vi "pump calibration.vi"(4 "pump ID":u8, 6 "pump cal command":T3=enum."Save default values", 8 "STAMP intercept":dbl, 9 "STAMP slope":dbl=2.52, 10 "flow rate":dbl[unit], 11 "Pump Calibration in":T1={"target 1"=0.0, "target 2"=0.0, "measured 1"=1e-06, "measured 2"=1e-06}) -> (0 "STAMP intercept out":dbl, 1 "STAMP slope out":dbl=2.52, 2 "modified flow rate":dbl[unit], 3 "Pump Calibration out":T1)   [LabVIEW 2010]
uses:
  calibration values.ctl
  calibration commands.ctl
  <vilib>/Utility/config.llb/Write Key (Double).vi
  <vilib>/Utility/config.llb/Read Key (Double).vi
  <vilib>/Utility/config.llb/NI_LVConfig.lvlib
panel:
  in  "pump calibrations default":T2(array[cluster])=[{"Pump Calibration"={"target 1"=0.0, "target 2"=1e-06, "measured 1"=0.0, "measured 2"=1e-06}, "STAMP slope"=1.0, "STAMP intercept"=0.0}, {"Pump Calibration"={"target 1"=0.0, "target 2"=1e-06, "measured 1"=0.0, "measured 2"=0.0}, "STAMP slope"=1.0, "STAMP intercept"=0.0}, {"Pump Calibration"={"target 1"=0.0, "target 2"=1e-06, "measured 1"=0.0, "measured 2"=0.0}, "STAMP slope"=1.0, "STAMP intercept"=0.0}, {"Pump Calibration"={"target 1"=0.0, "target 2"=1e-06, "measured 1"=0.0, "measured 2"=0.0}, "STAMP slope"=1.0, "STAMP intercept"=0.0}, {"Pump Calibration"={"target 1"=0.0, "target 2"=1e-06, "measured 1"=0.0, "measured 2"=0.0}, "STAMP slope"=1.0, "STAMP intercept"=0.0}, {"Pump Calibration"={"target 1"=0.0, "target 2"=1e-06, "measured 1"=0.0, "measured 2"=0.0}, "STAMP slope"=1.0, "STAMP intercept"=0.0}]
  out "pump calibrations":T2(array[cluster])
  in  "Pump Calibration default":T1={"target 1"=0.0, "target 2"=1e-06, "measured 1"=0.0, "measured 2"=1e-06}
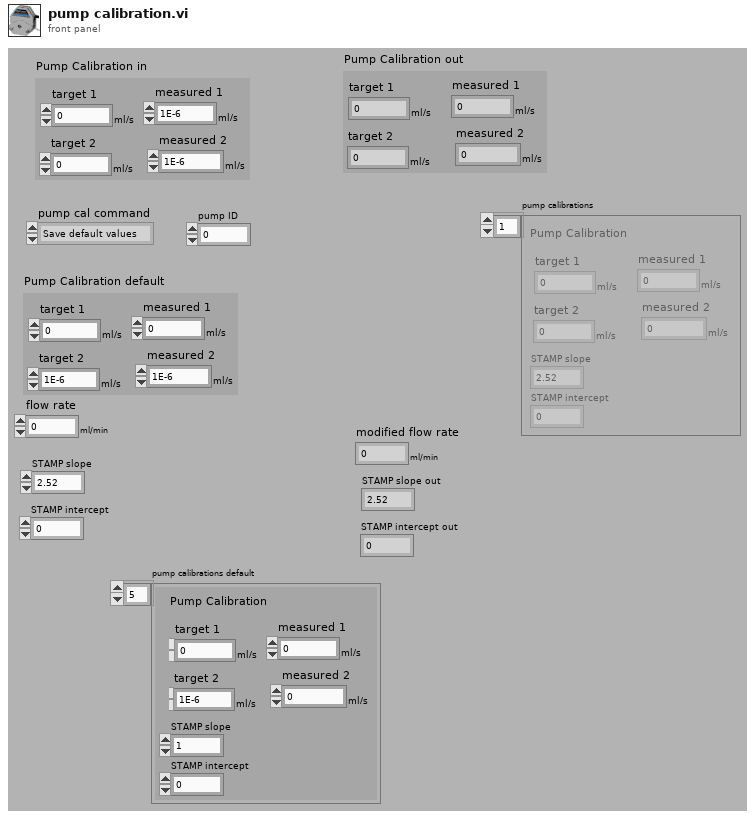
[diagram p1: front panel]
types:
  T1 = typedef "calibration values.ctl" = cluster{"target 1":dbl[unit], "target 2":dbl[unit], "measured 1":dbl[unit], "measured 2":dbl[unit]}
  T2 = cluster{"Pump Calibration":T1, "STAMP slope":dbl, "STAMP intercept":dbl}[]
  T3 = typedef "calibration commands.ctl" = enum16{"Get ini Path", "Save default values", "Save new calibration", "Read calibration", "Apply calibration", "Read STAMP mb", "Write STAMP mb"}
  T4 = typedef "NI_LVConfig.lvlib/Config Data RefNum.ctl" = refnum<k1>
  T5 = cluster{"Pump Calibration":T1, "STAMP slope":dbl, "STAMP intercept":dbl}
  T6 = cluster{"[0]":dbl[unit], "[1]":dbl[unit], "[2]":dbl[unit], "[3]":dbl[unit]}
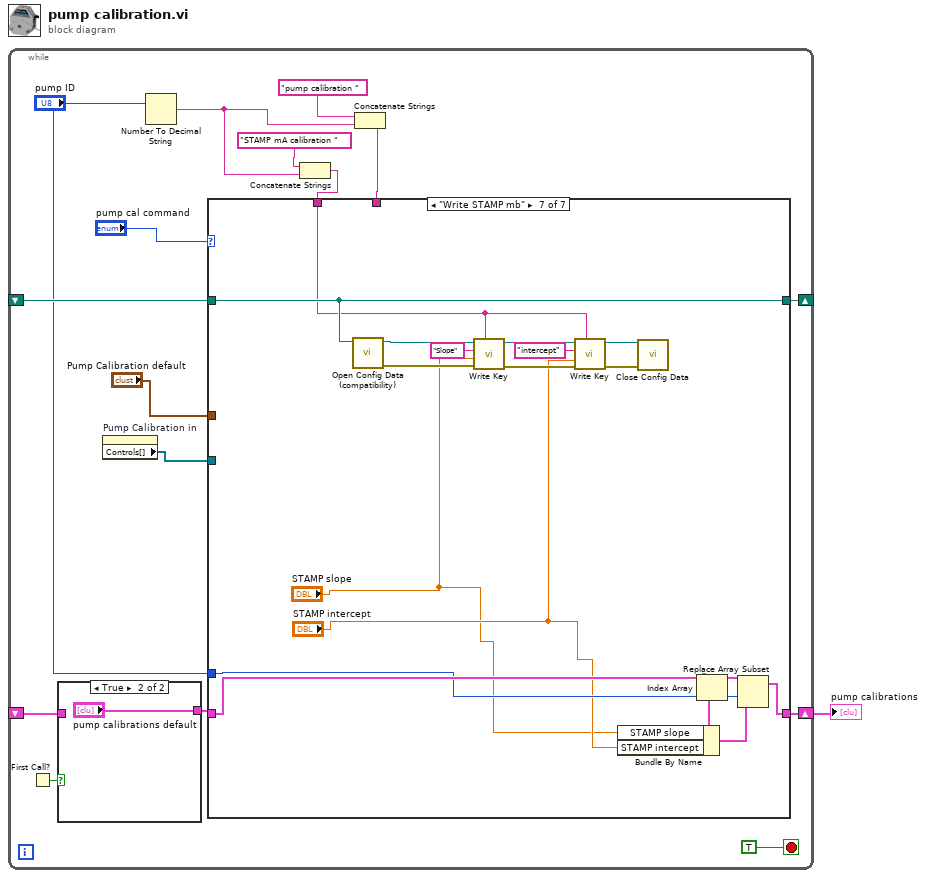
[diagram p0: block diagram]
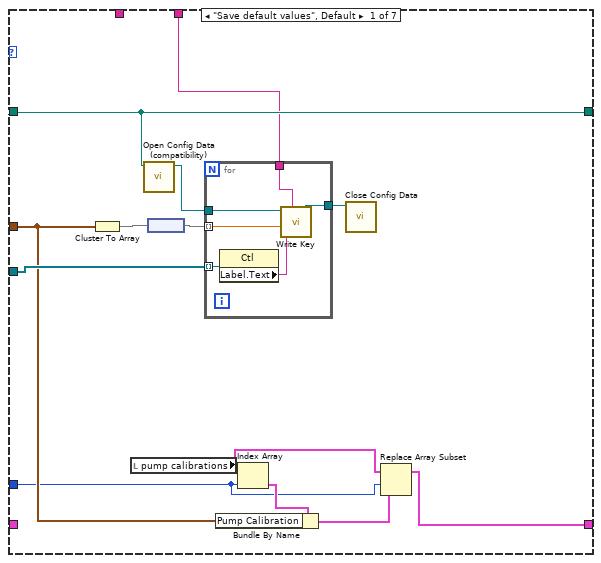
[diagram p3: hidden frame]
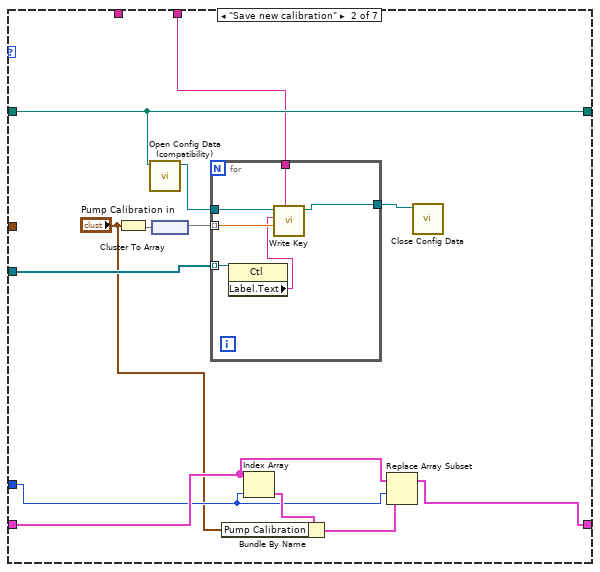
[diagram p4: hidden frame]
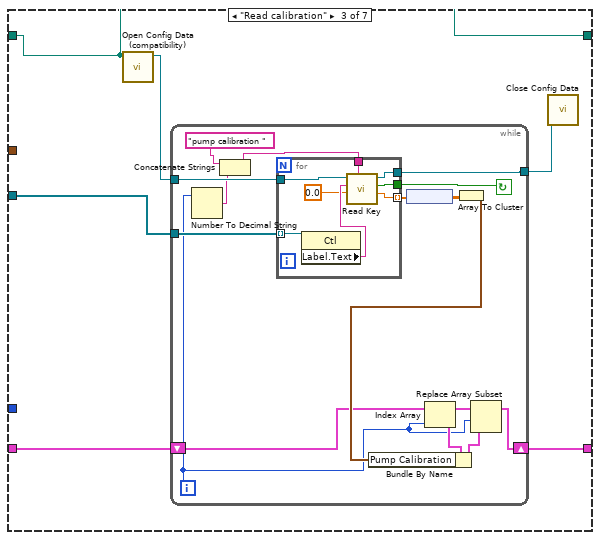
[diagram p5: hidden frame]
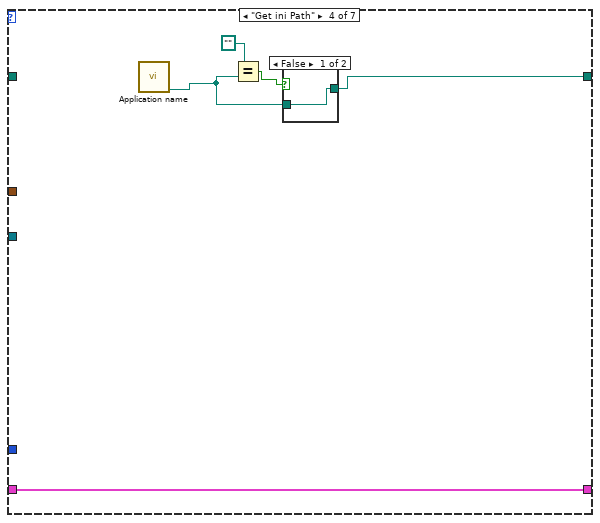
[diagram p6: hidden frame]
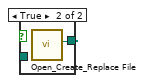
[diagram p7: hidden frame]
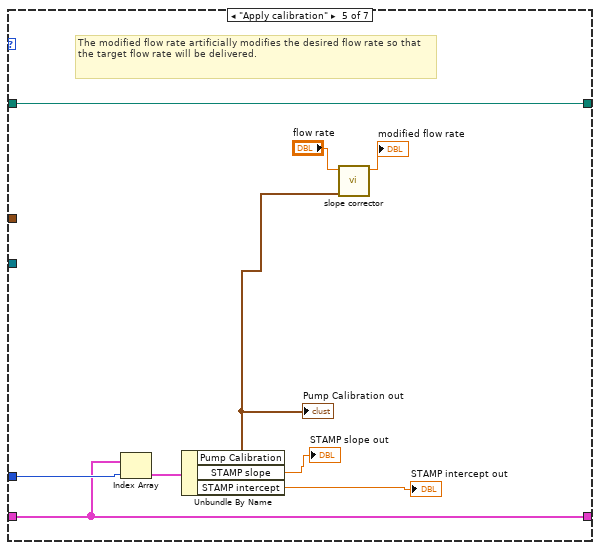
[diagram p8: hidden frame]
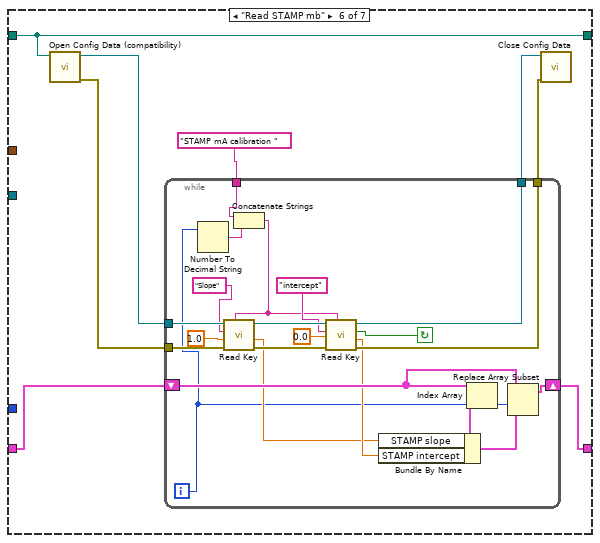
[diagram p9: hidden frame]
diagram:
  n1 = while {
    shift-right: [w14] -> _
    shift-left: _ -> [w16]
    shift-right: [w5] -> w1
    shift-left: _ -> [w3]
    stop <- TRUE stop-if-true
    n2 = First Call?() -> (First Call?: T/F=w4:bool)
    n3 = case shown="True" w4 {
      tunnel: w3 -> [w18 _]
      tunnel: [w18 "pump calibrations default"] -> w2
      frame False {
      }
      frame True {
      }
    }
    n4 = property on="Pump Calibration in" class="Clust (strict)"() -> ("Controls[]"=w15:refnum<vi>[])  [unwired: 2 in, 2 out]
    n5 = Number To Decimal String(number="pump ID") -> (decimal integer string=w8:string)  [unwired: 1 in]
    n6 = Concatenate Strings("STAMP mA calibration " ("section"), w8) -> (w7:string)
    n7 = Concatenate Strings("pump calibration " ("section"), w8) -> (w10:string)
    n8 = case shown="\"Write STAMP mb\"" "pump cal command" {
      tunnel: w16 -> [w29 w49 w60 _ w102 w110 w148]
      tunnel: w15 -> [w28 w48 w61 _ _ _ _]
      tunnel: [w29 w49 w60 w89 w102 w110 w148] -> w14
      tunnel: w7 -> [_ _ _ _ _ _ w139]
      tunnel: w10 -> [w26 w45 _ _ _ _ _]
      tunnel: "Pump Calibration default" -> [w24 _ _ _ _ _ _]
      tunnel: "pump ID" -> [w22 w40 _ _ w99 _ w134]
      tunnel: [w20 w42 w58 w87 w98 w104 w136] -> w5
      tunnel: w2 -> [_ w41 w59 w87 w98 w105 w135]
      frame "Save default values", Default {
        n9 = Cluster To Array(cluster=w24) -> (array=w31:dbl[unit][])
        n10 = local read "pump calibrations"() -> (w23:T2)
        n11 = call <vilib>:"Open Config Data (compatibility).vi"("configuration file path"=w29) -> ("refnum"=w32:T4)  [unwired: 8 in, 2 out]
        n12 = node(w31) -> (w27:dbl[])
        n13 = for {
          tunnel: w32 -> [w38]
          tunnel: w27 -> [w37] mode=indexing
          tunnel: w28 -> [w36] mode=indexing
          tunnel: w26 -> [w34]
          tunnel: [w33] -> w30
          n14 = property class="Ctl"(reference=w36) -> ("Label.Text"=w35:string)  [unwired: 1 in, 2 out]
          n15 = call-poly <vilib>:"Write Key.vi"("section"=w34, "value"=w37, "key"=w35, "refnum"=w38) -> ("refnum out"=w33:T4)  [unwired: 5 in, 2 out]
        }
        n16 = Index Array(array=w23, index=w22) -> (element=w25:T5)
        n17 = Bundle By Name(cluster=w25, "Pump Calibration"=w24) -> (w21:T5)
        n18 = call <vilib>:"Close Config Data.vi"("refnum"=w30) -> ()  [unwired: 9 in, 2 out]
        n19 = Replace Array Subset(array=w23, new element=w21, index=w22) -> (w20:T2)
      }
      frame "Save new calibration" {
        n20 = Cluster To Array(cluster="Pump Calibration in") -> (array=w46:dbl[unit][])
        n21 = call <vilib>:"Open Config Data (compatibility).vi"("configuration file path"=w49) -> ("refnum"=w51:T4)  [unwired: 8 in, 2 out]
        n22 = node(w46) -> (w47:dbl[])
        n23 = for {
          tunnel: w51 -> [w57]
          tunnel: w47 -> [w56] mode=indexing
          tunnel: w48 -> [w55] mode=indexing
          tunnel: w45 -> [w53]
          tunnel: [w52] -> w50
          n24 = property class="Ctl"(reference=w55) -> ("Label.Text"=w54:string)  [unwired: 1 in, 2 out]
          n25 = call-poly <vilib>:"Write Key.vi"("section"=w53, "value"=w56, "key"=w54, "refnum"=w57) -> ("refnum out"=w52:T4)  [unwired: 5 in, 2 out]
        }
        n26 = Index Array(array=w41, index=w40) -> (element=w44:T5)
        n27 = Bundle By Name(cluster=w44, "Pump Calibration"="Pump Calibration in") -> (w43:T5)
        n28 = Replace Array Subset(array=w41, new element=w43, index=w40) -> (w42:T2)
        n29 = call <vilib>:"Close Config Data.vi"("refnum"=w50) -> ()  [unwired: 9 in, 2 out]
      }
      frame "Read calibration" {
        n30 = call <vilib>:"Open Config Data (compatibility).vi"("configuration file path"=w60) -> ("refnum"=w63:T4)  [unwired: 8 in, 2 out]
        n31 = while {
          tunnel: w63 -> [w78]
          tunnel: [w77] -> w62
          tunnel: w61 -> [w75]
          shift-right: [w69] -> w58
          shift-left: w59 -> [w70]
          i -> [w64]
          stop <- w68 continue-if-true
          n32 = Number To Decimal String(number=w64) -> (decimal integer string=w66:string)  [unwired: 1 in]
          n33 = Concatenate Strings("pump calibration " ("section"), w66) -> (w65:string)
          n34 = for {
            tunnel: w78 -> [w86]
            tunnel: w75 -> [w85] mode=indexing
            tunnel: w65 -> [w83]
            tunnel: [w82] -> w77
            tunnel: [w80] -> w76 mode=indexing
            tunnel: [w79] -> w68
            n35 = property class="Ctl"(reference=w85) -> ("Label.Text"=w84:string)  [unwired: 1 in, 2 out]
            n36 = call-poly <vilib>:"Read Key.vi"("section"=w83, "default value"=0.0 ("target 1"), "key"=w84, "refnum"=w86) -> ("value"=w80:dbl, "found?"=w79:bool, "refnum out"=w82:T4)  [unwired: 4 in, 1 out]
          }
          n37 = node(w76) -> (w74:dbl[unit][])
          n38 = Index Array(array=w70, index=w64) -> (element=w73:T5)
          n39 = Array To Cluster(array=w74) -> (cluster=w71:T6)
          n40 = Bundle By Name(cluster=w73, "Pump Calibration"=w71) -> (w72:T5)
          n41 = Replace Array Subset(array=w70, new element=w72, index=w64) -> (w69:T2)
        }
        n42 = call <vilib>:"Close Config Data.vi"("refnum"=w62) -> ()  [unwired: 9 in, 2 out]
      }
      frame "Get ini Path" {
        n43 = call "Application name.vi"() -> ("Ini file path"=w88:path)  [unwired: 4 in, 3 out]
        n44 = Equal?(x=path "", y=w88) -> (x = y?=w91:bool)
        n45 = case shown="False" w91 {
          tunnel: [w92 w93] -> w89
          tunnel: w88 -> [w92 _]
          frame False {
          }
          frame True {
            n46 = call <vilib>:"Open_Create_Replace File.vi"() -> ("new file path"=w93:path)  [unwired: 8 in, 3 out]
          }
        }
      }
      frame "Apply calibration" {
        # "The modified flow rate artificially modifies the desired flow rate so that the target flow rate will be delivered."
        n47 = Index Array(array=w98, index=w99) -> (element=w97:T5)
        n48 = Unbundle By Name(w97) -> ("Pump Calibration"=w94:T1, "STAMP slope"=→"STAMP slope out":dbl, "STAMP intercept"=→"STAMP intercept out":dbl)
        "Pump Calibration out" <- w94
        n49 = call "slope corrector.vi"("Pump Calibration"=w94, "flow rate"="flow rate") -> ("modified flow rate"=→"modified flow rate":dbl[unit])  [unwired: 9 in]
      }
      frame "Read STAMP mb" {
        n50 = call <vilib>:"Open Config Data (compatibility).vi"("configuration file path"=w110) -> ("error out"=w107:errorcluster, "refnum"=w109:T4)  [unwired: 8 in, 1 out]
        n51 = while {
          tunnel: w109 -> [w131]
          tunnel: [w129] -> w108
          tunnel: w107 -> [w128]
          tunnel: [w126] -> w106
          shift-right: [w117] -> w104
          shift-left: w105 -> [w120]
          tunnel: "STAMP mA calibration " ("section") -> [w113]
          i -> [w111]
          stop <- w116 continue-if-true
          n52 = Number To Decimal String(number=w111) -> (decimal integer string=w112:string)  [unwired: 1 in]
          n53 = Concatenate Strings(w113, w112) -> (w114:string)
          n54 = call-poly <vilib>:"Read Key.vi"("section"=w114, "error in (no error)"=w128, "default value"=1.0 ("STAMP slope"), "key"="Slope", "refnum"=w131) -> ("error out"=w127:errorcluster, "value"=w118:dbl, "refnum out"=w130:T4)  [unwired: 3 in, 1 out]
          n55 = call-poly <vilib>:"Read Key.vi"("section"=w114, "error in (no error)"=w127, "default value"=0.0 ("STAMP intercept"), "key"="intercept", "refnum"=w130) -> ("error out"=w126:errorcluster, "value"=w119:dbl, "found?"=w116:bool, "refnum out"=w129:T4)  [unwired: 3 in]
          n56 = Index Array(array=w120, index=w111) -> (element=w122:T5)
          n57 = Bundle By Name(cluster=w122, "STAMP slope"=w118, "STAMP intercept"=w119) -> (w121:T5)
          n58 = Replace Array Subset(array=w120, new element=w121, index=w111) -> (w117:T2)
        }
        n59 = call <vilib>:"Close Config Data.vi"("error in (no error)"=w106, "refnum"=w108) -> ()  [unwired: 8 in, 2 out]
      }
      frame "Write STAMP mb" {
        n60 = call <vilib>:"Open Config Data (compatibility).vi"("configuration file path"=w148) -> ("error out"=w142:errorcluster, "refnum"=w147:T4)  [unwired: 8 in, 1 out]
        n61 = call-poly <vilib>:"Write Key.vi"("section"=w139, "error in (no error)"=w142, "value"="STAMP slope", "key"="Slope", "refnum"=w147) -> ("error out"=w141:errorcluster, "refnum out"=w146:T4)  [unwired: 4 in, 1 out]
        n62 = call-poly <vilib>:"Write Key.vi"("section"=w139, "error in (no error)"=w141, "value"="STAMP intercept", "key"="intercept", "refnum"=w146) -> ("error out"=w140:errorcluster, "refnum out"=w145:T4)  [unwired: 4 in, 1 out]
        n63 = call <vilib>:"Close Config Data.vi"("error in (no error)"=w140, "refnum"=w145) -> ()  [unwired: 8 in, 2 out]
        n64 = Index Array(array=w135, index=w134) -> (element=w138:T5)
        n65 = Bundle By Name(cluster=w138, "STAMP slope"="STAMP slope", "STAMP intercept"="STAMP intercept") -> (w137:T5)
        n66 = Replace Array Subset(array=w135, new element=w137, index=w134) -> (w136:T2)
      }
    }
  }
  "pump calibrations" <- w1
